vi "Host_Main.vi"() -> ()   [LabVIEW 2021]
uses:
  <vilib>/Utility/error.llb/DialogType.ctl
panel:
  in  "Stop Streaming":bool
  out "Numeric 2":i32
  out "Numeric":i32
  out "error out":errorcluster
  in  "Stream":bool
  in  "?":enum32{"Charts", "Raw Endevco", "Controller"}(tab)=enum."Raw Endevco"
  out "Size Array":i32[](array[numeric])
  out "?":dbl[][](graph)
  in  "X Scale.Range:Maximum RT":dbl=100000.0
  out "Waveform Chart":sgl[][](graph)
  in  "X Scale.Range:Maximum ESP":dbl
  in  "Tab Control":enum32{"Saving", "Parameters"}(tab)=enum."Parameters"
  in  "File name RT":string="RTData_20_03_Run1_TQC"
  in  "Path name RT":path=path "C:/Users/aabud/Desktop/Experiment_March_2023/Saved Data"
  out "AI_Filename":string
  in  "Start Logging":bool
  in  "Save Data":bool
  in  "File name ESP":string="ESPData_20_03_Run1_TQC"
  in  "Path name  ESP":path=path "C:/Users/aabud/Desktop/Experiment_March_2023/Saved Data"
  out "start saving esp":bool
  out "ESP_FileName":string
  out "Stream on?":string
  # "Time  Critical Loop"
  # "Non  Critical Loop"
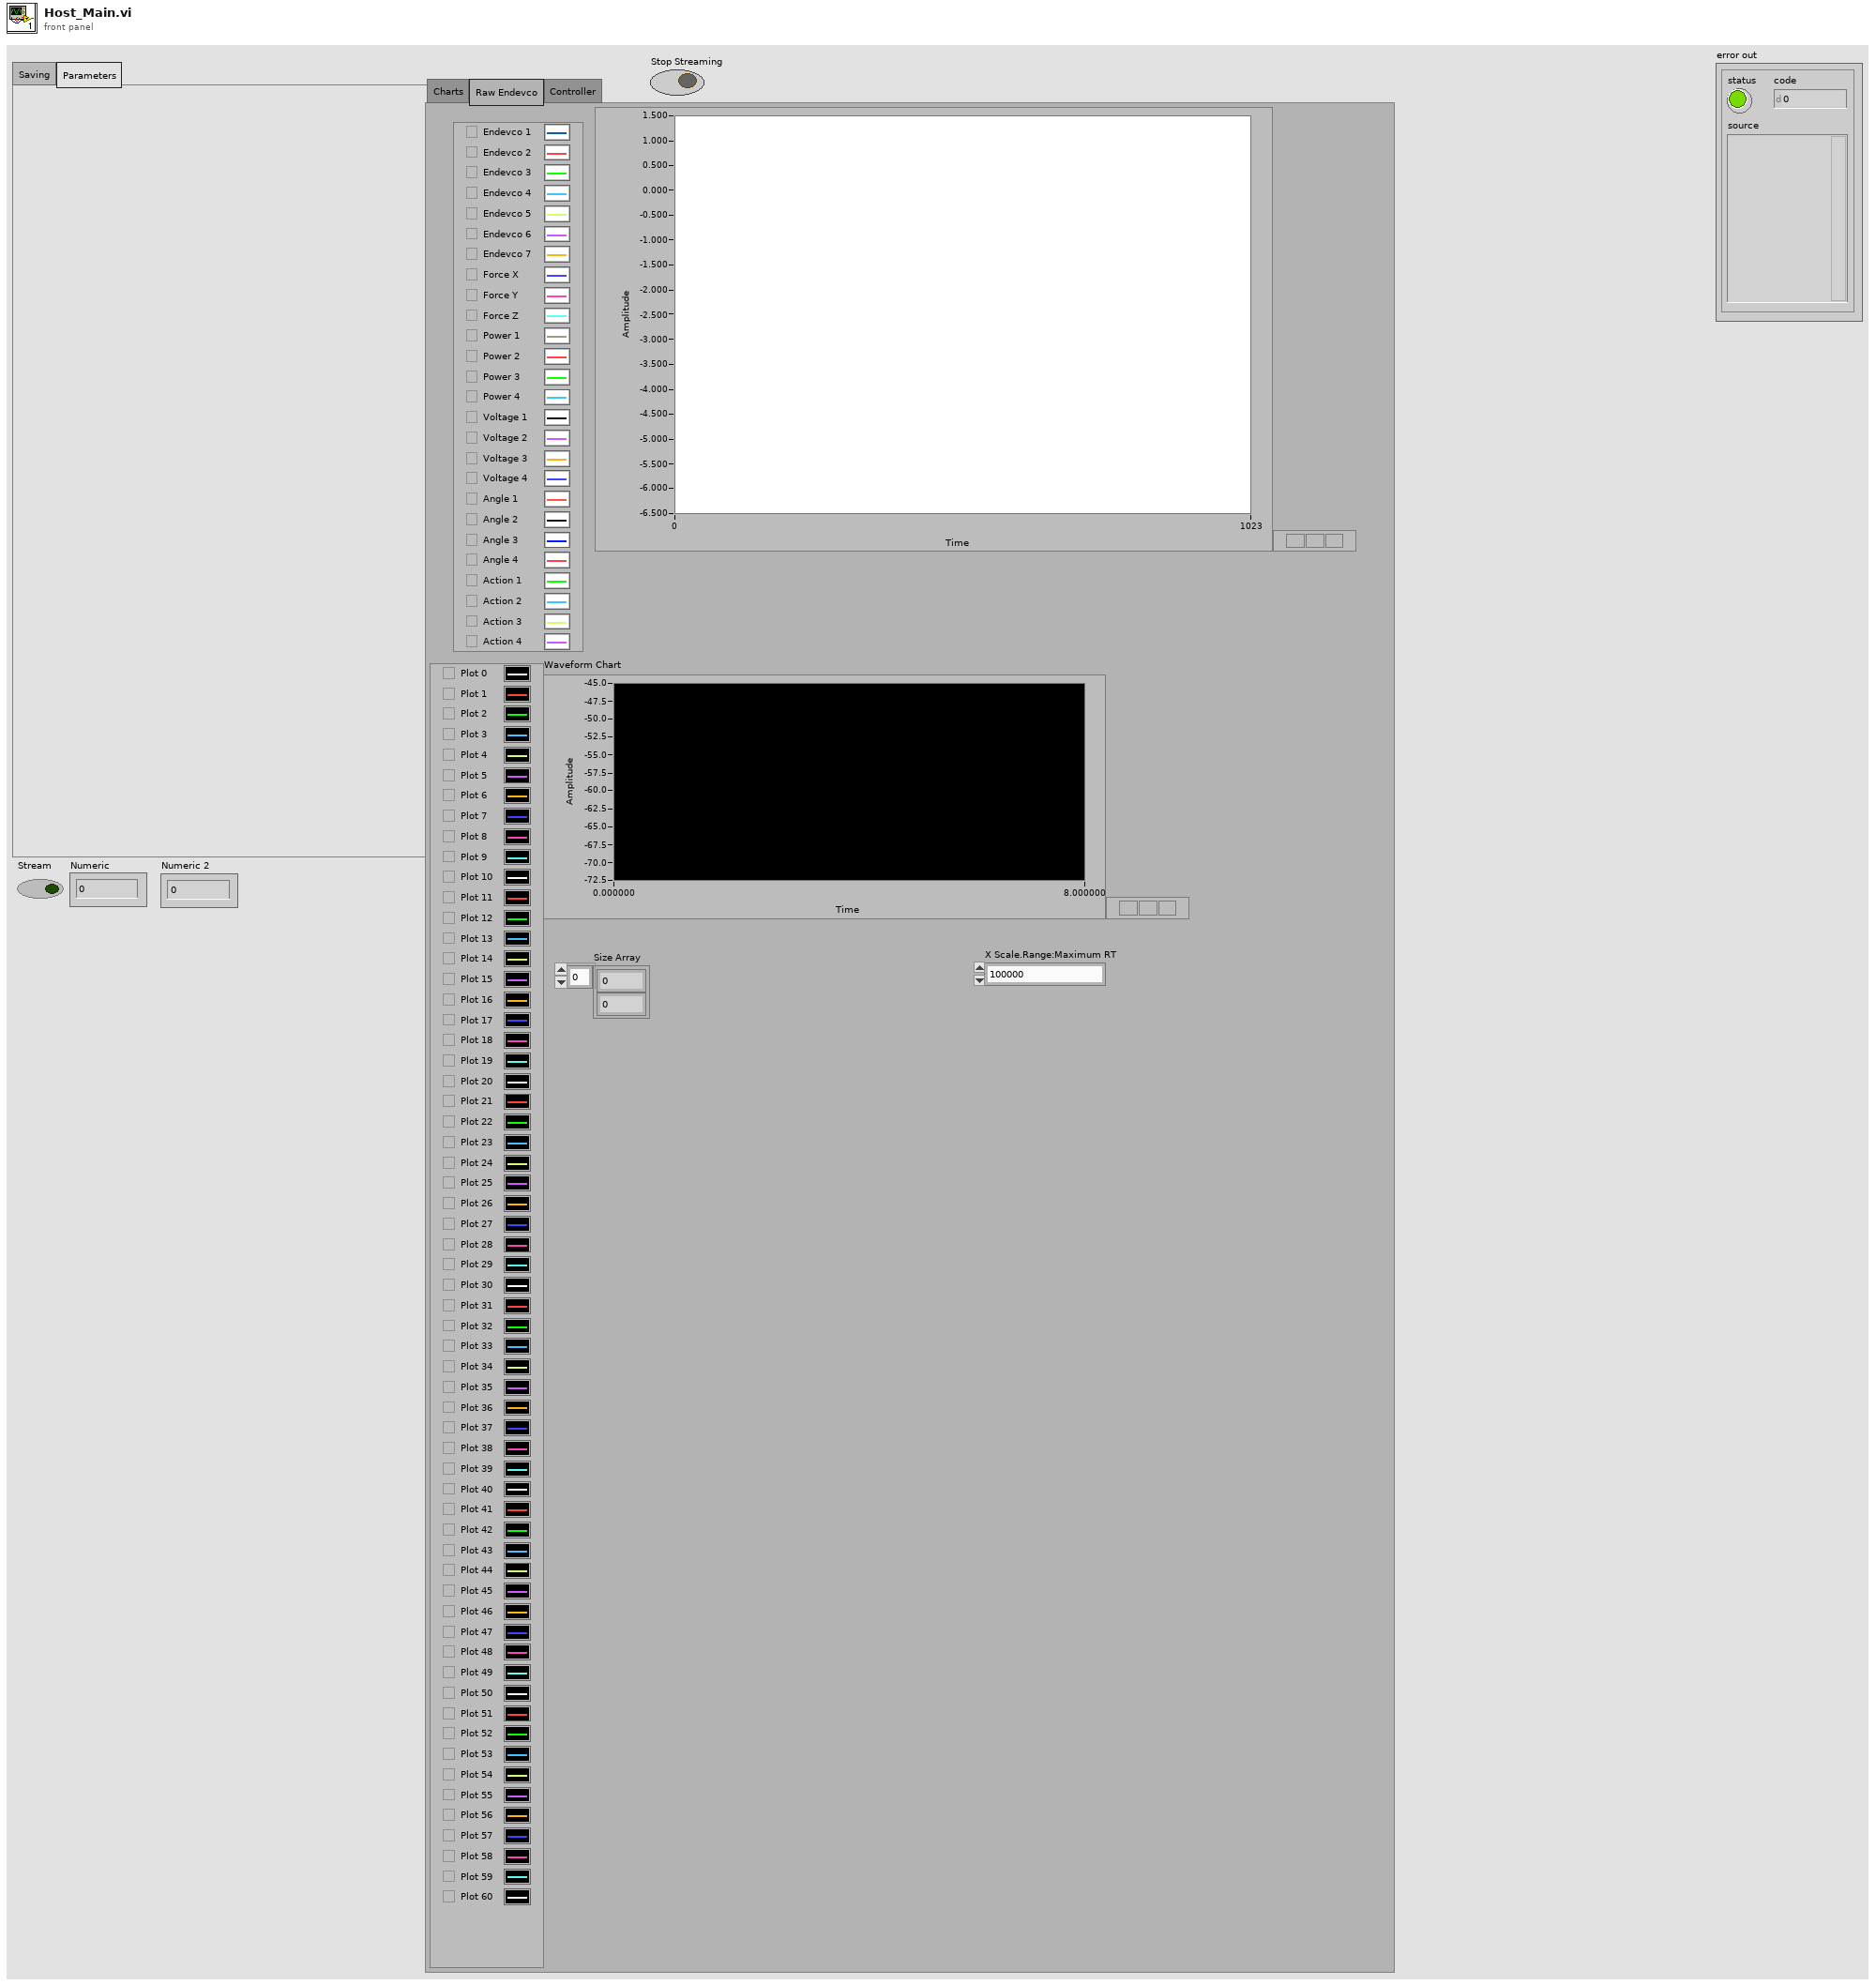
[diagram p1: front panel]
types:
  T1 = enum16{"Standard", "Buffered", "CRLF", "Immediate"}
  T2 = typedef "DialogType.ctl" = u16
  T3 = enum16{"big-endian, network order", "native, host order", "little-endian"}
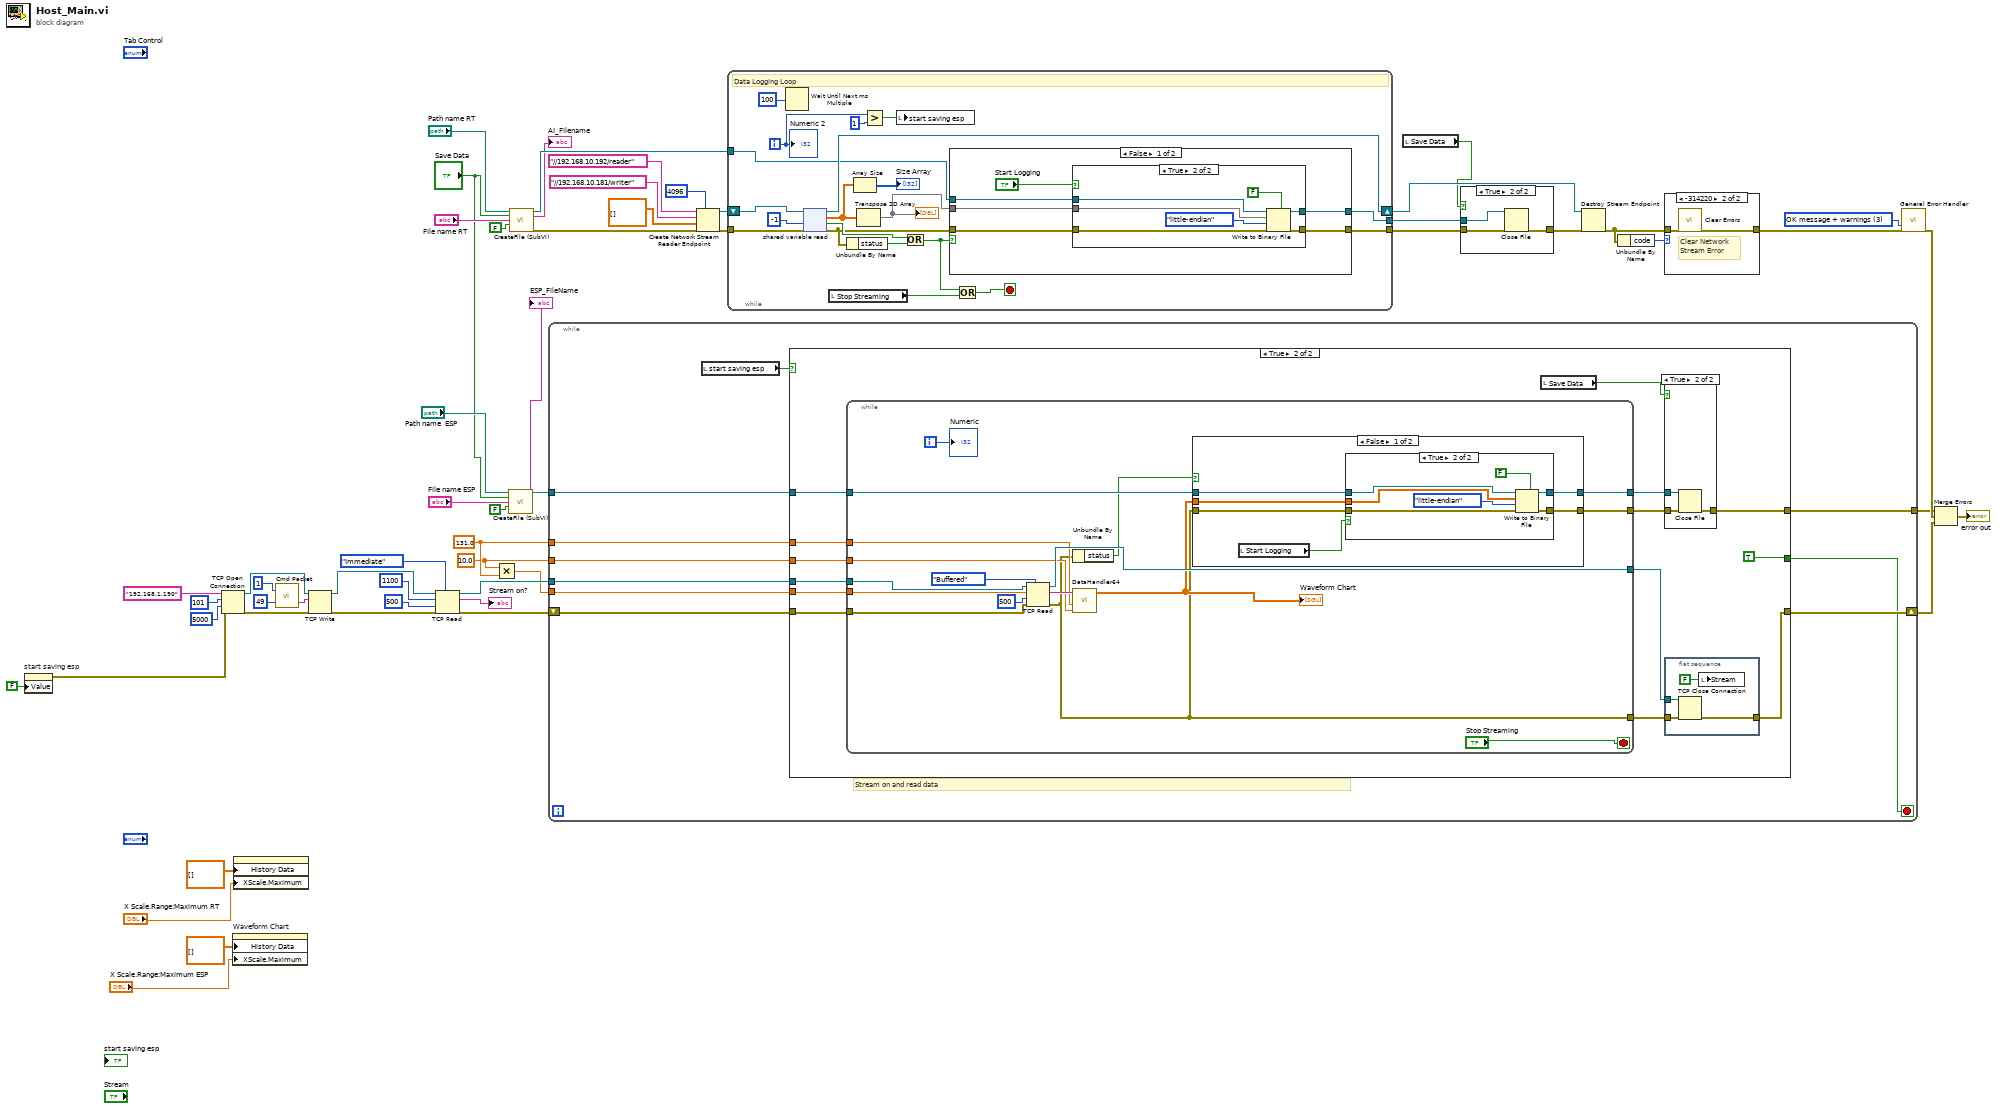
[diagram p0: block diagram]
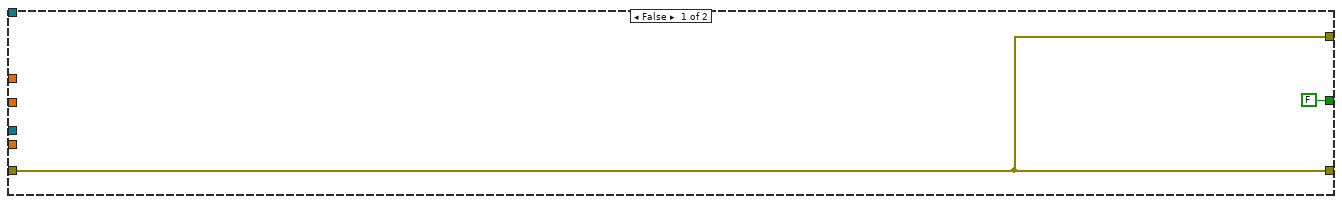
[diagram p2: hidden frame]
diagram:
  w18 = 10.0 ("Sampling Rate")
  w19 = 131.0 ("y")
  w51 = T2 3 items=["no dialog", "OK message", "continue or stop message", "OK message + warnings", "continue/stop + warnings"] ("type of dialog (OK msg:1)")
  n1 = property on="start saving esp" class="Bool (strict)"("Value"=FALSE ("start saving esp")) -> (error out=w1:errorcluster)  [unwired: 2 in, 1 out]
  n2 = TCP Open Connection(address="192.168.1.190", remote port or service name=u16 101 ("Port"), timeout ms (60000)=5000, error in (no error)=w1) -> (connection ID=w27:refnum<k5>, error out=w17:errorcluster)  [unwired: 1 in]
  n3 = property on="Waveform Chart" class="WFChart (strict)"("History Data"=sgl[][] [], "XScale.Maximum"="X Scale.Range:Maximum ESP") -> ()  [unwired: 2 in, 2 out]
  n4 = property class="WFChart (strict)"("History Data"=dbl[][] [], "XScale.Maximum"="X Scale.Range:Maximum RT") -> ()  [unwired: 2 in, 2 out]
  n5 = call "Cmd Packet.vi"("Command Byte"=49 ("data in"), "Parameter Byte"=1 ("data in")) -> ("Command Packet Byte String"=w31:string)  [unwired: 1 out]
  n6 = TCP Write(connection ID=w27, data in=w31, error in (no error)=w17) -> (connection ID out=w29:refnum<k5>, error out=w16:errorcluster)  [unwired: 1 in, 1 out]
  n7 = TCP Read(connection ID=w29, bytes to read=1100, error in (no error)=w16, 7:T1."Immediate" ("mode (standard)"), 9:500 ("timeout ms (25000)")) -> (connection ID out=w32:refnum<k5>, data out=→"Stream on?":string, error out=w15:errorcluster)
  n8 = Multiply(x=w18, y=w19) -> (x*y=w28:dbl)
  n9 = call "CreateFile (SubVI).vi"("Path name"="Path name  ESP", "Save Data"="Save Data", "File name"="File name ESP", "Date Folder"=FALSE) -> ("Byte Stream File out"=w9:refnum<file>, "String"=→"ESP_FileName":string)  [unwired: 9 in, 1 out]
  n10 = call "CreateFile (SubVI).vi"("Path name"="Path name RT", "Save Data"="Save Data", "File name"="File name RT", "Date Folder"=FALSE) -> ("Byte Stream File out"=w48:refnum<file>, "String"=→"AI_Filename":string, "error out"=w37:errorcluster)  [unwired: 9 in]
  n11 = while {
    tunnel: w32 -> [w66]
    tunnel: w28 -> [w65]
    tunnel: w19 -> [w64]
    tunnel: w18 -> [w63]
    shift-right: [w60] -> w13
    shift-left: w15 -> [w62]
    tunnel: w9 -> [w59]
    tunnel: [w58] -> w8
    stop <- w57 stop-if-true
    # "Stream on and read data"
    n12 = local read "start saving esp"() -> (w61:bool)
    n13 = case shown="True" w61 {
      tunnel: w66 -> [_ w82]
      tunnel: w65 -> [_ w81]
      tunnel: w64 -> [_ w80]
      tunnel: w63 -> [_ w79]
      tunnel: w62 -> [w68 w78]
      tunnel: [w68 w77] -> w60
      tunnel: w59 -> [_ w75]
      tunnel: [w68 w70] -> w58
      tunnel: [FALSE TRUE] -> w57
      frame False {
      }
      frame True {
        n14 = while {
          tunnel: [w104] -> w76
          tunnel: w82 -> [w100]
          tunnel: w81 -> [w103]
          tunnel: w80 -> [w102]
          tunnel: w79 -> [w101]
          tunnel: w78 -> [w99]
          tunnel: [w94] -> w73
          tunnel: w75 -> [w96]
          tunnel: [w93] -> w72
          tunnel: [w92] -> w71
          i -> [w98]
          stop <- "Stop Streaming" stop-if-true
          n15 = TCP Read(connection ID=w100, bytes to read=w103, error in (no error)=w99, 7:T1."Buffered" ("mode (standard)"), 9:500 ("timeout ms (25000)")) -> (connection ID out=w104:refnum<k5>, data out=w107:string, error out=w92:errorcluster)
          n16 = Unbundle By Name(w92) -> ("status"=w95:bool)
          n17 = call "DataHandler64.vi"("Data Cycles Per Buffer"=w101, "Rx Packet Byte size"=w102, "data out"=w107) -> ("Data"=w97:sgl[][])  [unwired: 2 in, 4 out]
          "Waveform Chart" <- w97
          n18 = case shown="False" w95 {
            tunnel: w97 -> [w110 _]
            tunnel: w96 -> [w113 w124]
            tunnel: [w112 w124] -> w93
            tunnel: [w111 w123] -> w94
            tunnel: w92 -> [w108 w123]
            frame False {
              n19 = local read "Start Logging"() -> (w109:bool)
              n20 = case shown="True" w109 {
                tunnel: w113 -> [w115 w122]
                tunnel: [w115 w121] -> w112
                tunnel: [w114 w120] -> w111
                tunnel: w110 -> [_ w119]
                tunnel: w108 -> [w114 w116]
                frame False {
                }
                frame True {
                  n21 = Write to Binary File(file (use dialog)=w122, data=w119, error in=w116, 5:FALSE ("prepend array or string size? (T)"), 9:T3."little-endian" ("byte order (0:big-endian, network order)")) -> (refnum out=w121:refnum<file>, error out=w120:errorcluster)  [unwired: 1 in, 1 out]
                }
              }
            }
            frame True {
            }
          }
          "Numeric" <- w98
        }
        n22 = local read "Save Data"() -> (w74:bool)
        n23 = case shown="True" w74 {
          tunnel: w72 -> [_ w86]
          tunnel: w73 -> [w83 w85]
          tunnel: [w83 w84] -> w70
          frame False {
          }
          frame True {
            n24 = Close File(refnum=w86, error in=w85) -> (error out=w84:errorcluster)  [unwired: 1 out]
          }
        }
        n25 = flat-sequence {
          tunnel: [w89] -> w77
          tunnel: w71 -> [w88]
          tunnel: w76 -> [w87]
          frame #0 {
            n26 = TCP Close Connection(connection ID=w87, error in (no error)=w88) -> (error out=w89:errorcluster)  [unwired: 1 in, 1 out]
            n27 = local write "Stream"(FALSE) -> ()
          }
        }
      }
    }
  }
  n28 = Create Network Stream Reader Endpoint(7:4096 ("reader buffer size"), 8:w37, 9:dbl[][] [], 10:"//192.168.10.181/writer" ("writer url"), 11:"//192.168.10.192/reader" ("reader name")) -> (0:w39:errorcluster, 3:w43:refnum<k21>)  [unwired: 2 in]
  n29 = while {
    shift-right: [w143] -> w56
    shift-left: w43 -> [w144]
    tunnel: w39 -> [w133]
    tunnel: w48 -> [w139]
    tunnel: [w138] -> w47
    tunnel: [w137] -> w46
    i -> [w128]
    stop <- w136 stop-if-true
    # "Data Logging Loop"
    n30 = Wait Until Next ms Multiple(millisecond multiple=u32 100) -> ()  [unwired: 1 out]
    n31 = shared-variable-read(w144, w133, -1 ("timeout ms (-1)")) -> (w143:refnum<k21>, w131:errorcluster, w140:bool, w130:dbl[][])
    n32 = local read "Stop Streaming"() -> (w125:bool)
    n33 = Unbundle By Name(w131) -> ("status"=w135:bool)
    n34 = Array Size(array=w130) -> (size(s)=→"Size Array":i32[])
    n35 = Transpose 2D Array(2D array=w130) -> (transposed array=w129:dbl[][])
    "?" <- w129
    n36 = Greater?(x=w128, y=1) -> (0:w126:bool)
    n37 = local write "start saving esp"(w126) -> ()
    n38 = Or(x=w140, y=w135) -> (x .or. y?=w132:bool)
    n39 = case shown="False" w132 {
      tunnel: w129 -> [w147 _]
      tunnel: w139 -> [w150 w161]
      tunnel: [w149 w161] -> w138
      tunnel: w131 -> [w146 w160]
      tunnel: [w148 w160] -> w137
      frame False {
        n40 = case shown="True" "Start Logging" {
          tunnel: w150 -> [w152 w159]
          tunnel: [w152 w158] -> w149
          tunnel: w146 -> [w151 w157]
          tunnel: [w151 w156] -> w148
          tunnel: w147 -> [_ w155]
          frame False {
          }
          frame True {
            n41 = Write to Binary File(file (use dialog)=w159, data=w155, error in=w157, 5:FALSE ("prepend array or string size? (T)"), 9:T3."little-endian" ("byte order (0:big-endian, network order)")) -> (refnum out=w158:refnum<file>, error out=w156:errorcluster)  [unwired: 1 in, 1 out]
          }
        }
      }
      frame True {
      }
    }
    n42 = Or(x=w132, y=w125) -> (x .or. y?=w136:bool)
    "Numeric 2" <- w128
  }
  n43 = local read "Save Data"() -> (w36:bool)
  n44 = case shown="True" w36 {
    tunnel: w47 -> [_ w165]
    tunnel: w46 -> [w162 w164]
    tunnel: [w162 w163] -> w38
    frame False {
    }
    frame True {
      n45 = Close File(refnum=w165, error in=w164) -> (error out=w163:errorcluster)  [unwired: 1 out]
    }
  }
  n46 = Destroy Stream Endpoint(8:w38, 11:w56) -> (0:w50:errorcluster)
  n47 = Unbundle By Name(w50) -> ("code"=w49:i32)
  n48 = case shown="-314220" w49 {
    tunnel: w50 -> [w166 w168]
    tunnel: [w166 w167] -> w40
    frame 0, Default {
    }
    frame -314220 {
      # "Clear Network \nStream Error"
      n49 = call <vilib>:"Clear Errors.vi"("error in (no error)"=w168) -> ("error out"=w167:errorcluster)  [unwired: 5 in, 1 out]
    }
  }
  n50 = call <vilib>:"General Error Handler.vi"("type of dialog (OK msg:1)"=w51, "error in (no error)"=w40) -> ("error out"=w33:errorcluster)  [unwired: 9 in, 4 out]
  n51 = Merge Errors(w8, w33, w13) -> (→"error out":errorcluster)
